vi "Offset and Multiplier to Array.vi"(1 "Size":i32, 2 "Offset and Multiplier":T1) -> (0 "Array":dbl[](array[numeric]))   [LabVIEW 2016, in "graph_utilities.lvlib"]
uses:
  <vilib>/Utility/miscctls.llb/LVOffsetAndMultiplierTypeDef.ctl
  graph_utilities.lvlib
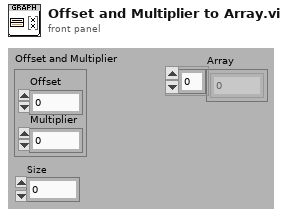
[diagram p1: front panel]
types:
  T1 = typedef "LVOffsetAndMultiplierTypeDef.ctl" = cluster{"Offset":dbl, "Multiplier":dbl}
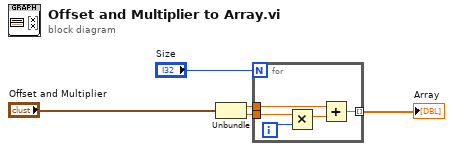
[diagram p0: block diagram]
diagram:
  n1 = Unbundle("Offset and Multiplier") -> ("Offset"=w1:dbl, "Multiplier"=w2:dbl)
  n2 = for {
    N: "Size" -> [_]
    tunnel: w1 -> [w8]
    tunnel: w2 -> [w10]
    tunnel: [w6] -> w5 mode=indexing
    i -> [w9]
    n3 = Multiply(x=w10, y=w9) -> (x*y=w7:dbl)
    n4 = Add(x=w8, y=w7) -> (x+y=w6:dbl)
  }
  "Array" <- w5
